vi "Start Multiple Listen.vi"(8 "error in (no error)":errorcluster, 10 "Functions":string[](array[string]), 11 "input in":refnum<class "input.lvclass">) -> (0 "error out":errorcluster, 3 "input out":refnum<class "input.lvclass">)   [LabVIEW 2015, in "input.lvclass"]
uses:
  input.lvclass
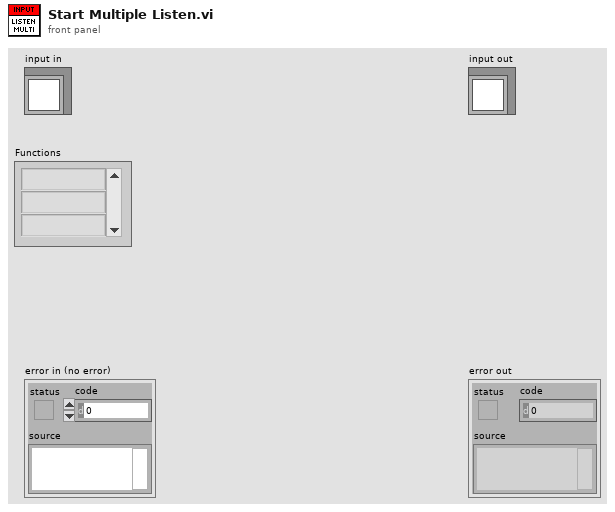
[diagram p1: front panel]
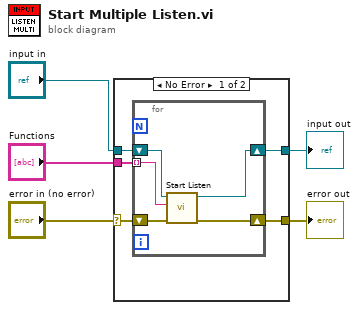
[diagram p0: block diagram]
diagram:
  n1 = case shown="No Error" "error in (no error)" {
    selector: "error in (no error)" -> [w10 w17]
    tunnel: [w8 w17] -> w4
    tunnel: [w7 w16] -> w2
    tunnel: "input in" -> [w9 w16]
    tunnel: "Functions" -> [w6 _]
    frame No Error {
      n2 = for {
        shift-right: [w14] -> w7
        shift-left: w9 -> [w15]
        shift-right: [w12] -> w8
        shift-left: w10 -> [w13]
        tunnel: w6 -> [w11] mode=indexing
        n3 = call "Start Listen.vi"("error in (no error)"=w13, "Function"=w11, "input in"=w15) -> ("error out"=w12:errorcluster, "input out"=w14:refnum<class "input.lvclass">)  [unwired: 7 in]
      }
    }
    frame Error {
    }
  }
  "error out" <- w4
  "input out" <- w2
